vi "ps5000a acquire GEECS.vi"(8 "error in (no error)":errorcluster, 11 "picoscope in":refnum<class "picoscope.lvclass">) -> (0 "error out":errorcluster, 1 "GEECS waveforms info":T3(array[cluster]), 2 "TraceGUI-Info":T2, 3 "scope traces":i16[][](array[numeric]), 4 "Channel A Settings":T1, 5 "Waveform Data":waveform(dbl)[](graph))   [LabVIEW 2020, in "picoscope.lvclass"]
uses:
  picoscope.lvclass
  Shared/TraceGUI-Info.ctl
  picoscope.lvclass/picoscope.ctl
panel:
  out "Channel B Settings":T1
  out "tme (ms)":u32
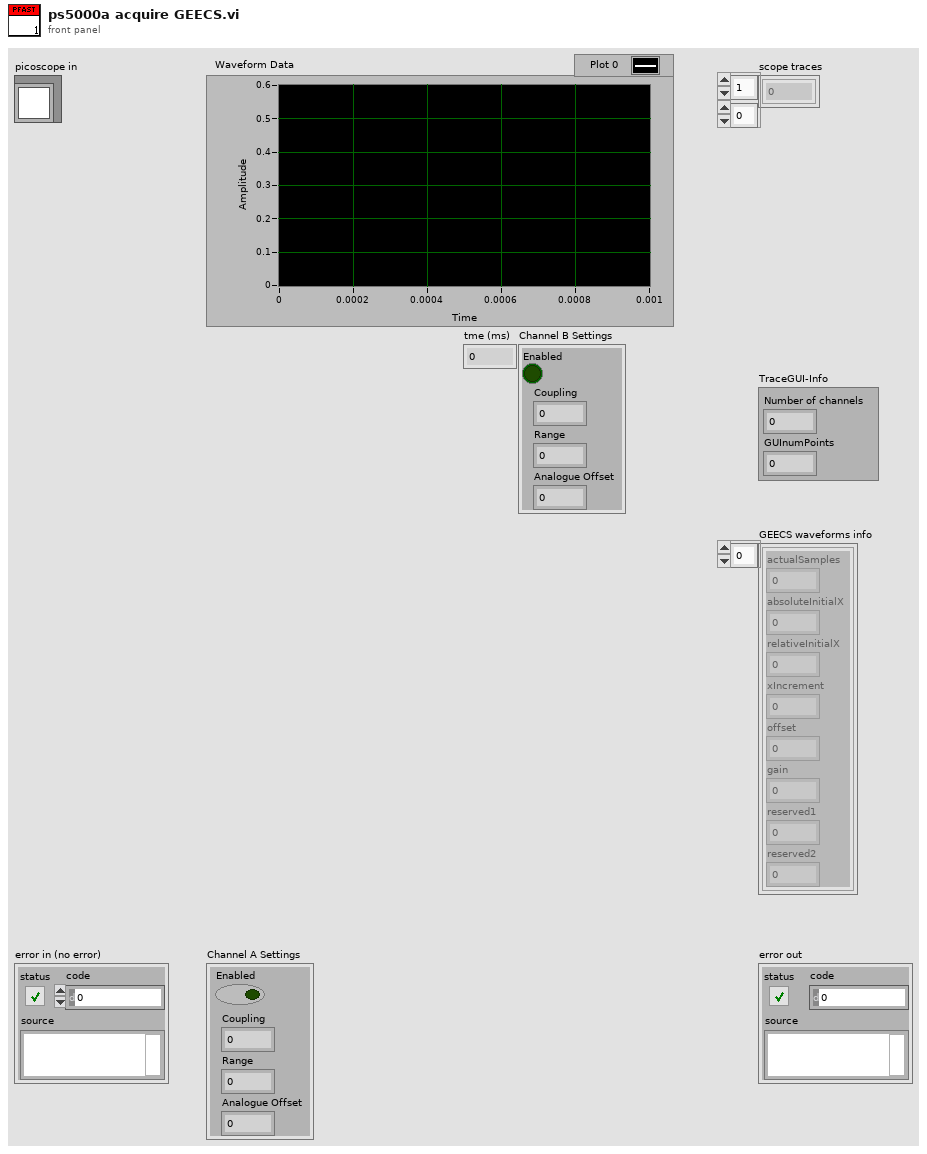
[diagram p1: front panel]
types:
  T1 = cluster{"Enabled":bool, "Coupling":i16, "Range":u16, "Analogue Offset":sgl}
  T2 = typedef "TraceGUI-Info.ctl" = cluster{"Number of channels":dbl, "GUInumPoints":i32}
  T3 = cluster{"actualSamples":i32, "absoluteInitialX":dbl, "relativeInitialX":dbl, "xIncrement":dbl, "offset":dbl, "gain":dbl, "reserved1":dbl, "reserved2":dbl}[]
  T4 = cluster{"Driver Version":string, "USB Version":string, "Hardware":string, "Variant":string, "Batch and Serial":string, "Cal Date":string, "Kernel Version":string, "Digital HW Version":string, "Analogue HW Version":string, "MSO":bool, "Number of channels":i16}
  T5 = cluster{"preTriggerSamples":u32, "postTriggerSamples":u32, "timebase":u32, "Down-Sample Mode":i32, "Down Sample Ratio":u32, "Number of Captures":u32}
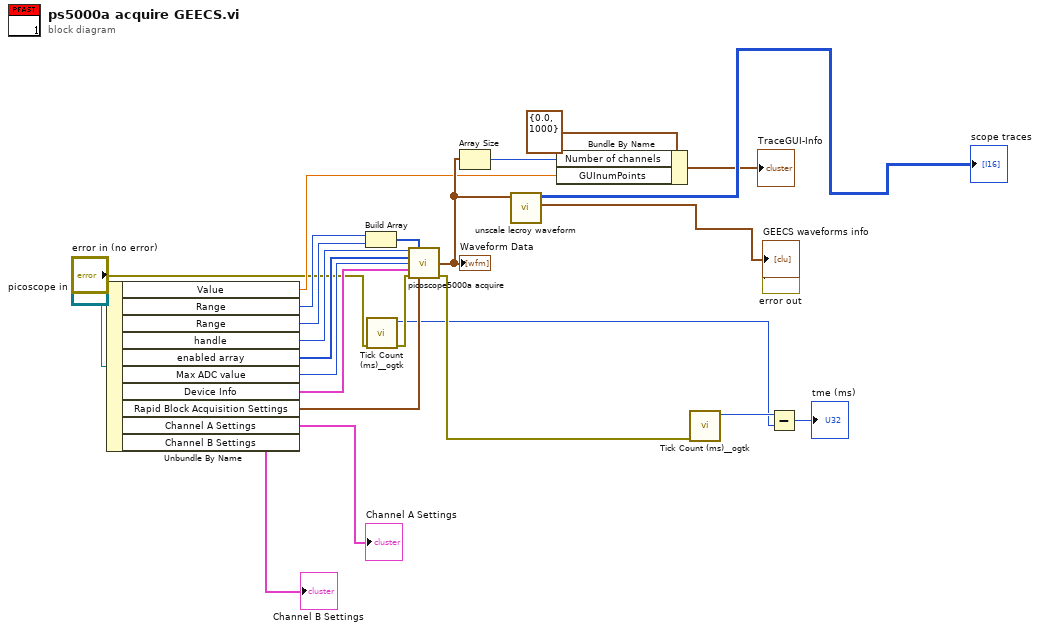
[diagram p0: block diagram]
diagram:
  n1 = Unbundle By Name("picoscope in") -> ("Value"=w12:dbl, "Range"=w17:u16, "Range"=w18:u16, "handle"=w13:i16, "enabled array"=w21:i16[], "Max ADC value"=w14:i16, "Device Info"=w15:T4, "Rapid Block Acquisition Settings"=w19:T5, "Channel A Settings"=→"Channel A Settings":T1, "Channel B Settings"=→"Channel B Settings":T1)
  n2 = Build Array(w17, w18) -> (w22:u16[])
  n3 = call <userlib>:"Tick Count (ms)__ogtk.vi"("error in (no error)"="error in (no error)") -> ("error out"=w6:errorcluster, "millisecond timer value"=w3:u32)  [unwired: 9 in]
  n4 = call "picoscope5000a acquire.vi"("handle in"=w13, "Ranges"=w22, "enabled array"=w21, "Max ADC value"=w14, "Device Info"=w15, "error in (no error)"=w6, "Rapid Block Acquisition Settings"=w19) -> ("Waveform Data"=w16:waveform(dbl)[], "error out"=w5:errorcluster)  [unwired: 4 in, 3 out]
  "Waveform Data" <- w16
  n5 = Array Size(array=w16) -> (size(s)=w10:i32)
  n6 = call "unscale lecroy waveform.vi"("Waveform Data"=w16) -> ("GEECS waveforms info"=→"GEECS waveforms info":T3, "scope traces"=→"scope traces":i16[][])  [unwired: 9 in]
  n7 = Bundle By Name(cluster=T2 {"Number of channels"=0.0, "GUInumPoints"=1000} ("TraceGUI-Info"), "Number of channels"=w10, "GUInumPoints"=w12) -> (→"TraceGUI-Info":T2)
  n8 = call <userlib>:"Tick Count (ms)__ogtk.vi"("error in (no error)"=w5) -> ("millisecond timer value"=w4:u32)  [unwired: 9 in, 1 out]
  n9 = Subtract(x=w4, y=w3) -> (x-y=→"tme (ms)":u32)
